vi "Inst.TC.Create.vi"(8 "error in (no error)":errorcluster, 11 "Inst.TC in":refnum<class "Inst.TC.lvclass">) -> (0 "error out":errorcluster, 2 "Inst.TC Public Events":T1, 3 "Inst.TC out":refnum<class "Inst.TC.lvclass">)   [LabVIEW 2019, in "Inst.TC.lvclass"]
uses:
  Inst.TC.lvclass
  C:/Program Files (x86)/National Instruments/LabVIEW 2019/user.lib/LevyLab/Instrument Framework/Instrument/Instrument.lvclass
  C:/Program Files (x86)/National Instruments/LabVIEW 2019/vi.lib/JKI/JKI SMO/SMO/SMO.lvclass
  Typedefs/PublicEvents--Cluster.ctl
  Typedefs/PublicEvents--Inst.TC.MessageFromProcess.ctl
  <userlib>/LevyLab/RemoteControl/RemoteControl/Typedefs/Message--Cluster.ctl
  <vilib>/JKI/JKI SMO/SMO/Typedefs/SMOState --Enum.ctl
  Inst.TC.lvclass/Inst.TC.ctl
  <vilib>/JKI/JKI SMO/SMO/SMO.lvclass
  <userlib>/LevyLab/Instrument Framework/Instrument/Instrument.lvclass
  FP-TC-Shared/FP-TC-Shared.lvclass
  <userlib>/LevyLab/RemoteControl/RemoteControl/RemoteControl.lvclass
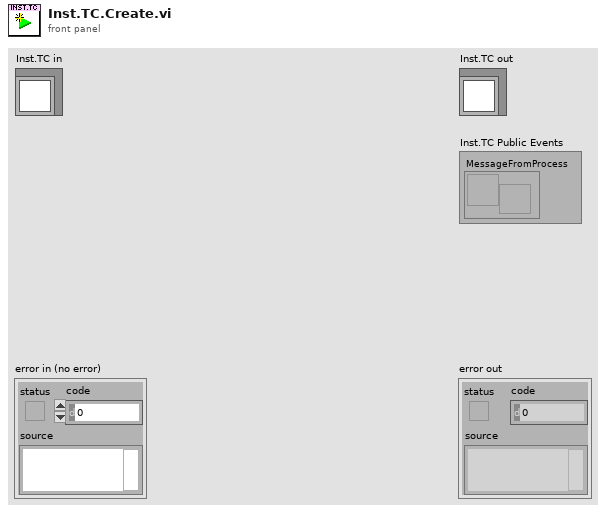
[diagram p1: front panel]
types:
  T1 = typedef "Inst.TC.lvclass/PublicEvents--Cluster.ctl" = cluster{"MessageFromProcess":refnum<user-event>}
  T2 = typedef "SMO.lvclass/SMOState --Enum.ctl" = enum16{"unknown", "Created", "Started", "Stopped"}
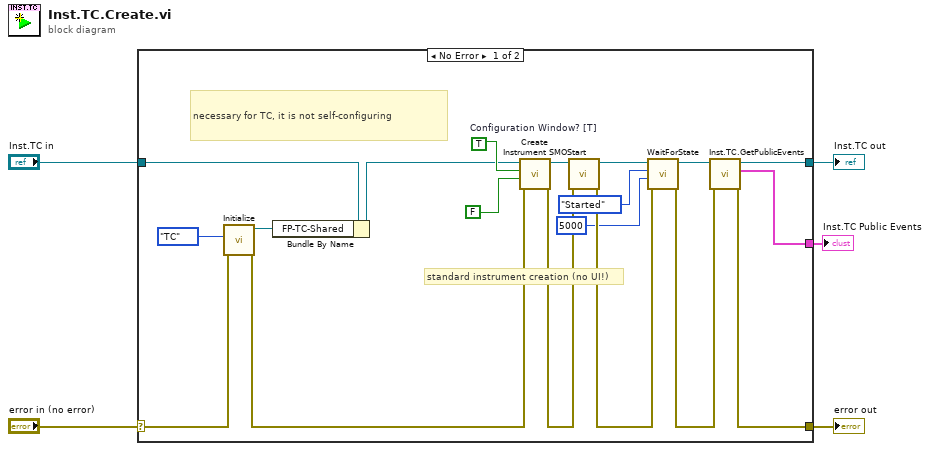
[diagram p0: block diagram]
diagram:
  n1 = case shown="No Error" "error in (no error)" {
    selector: "error in (no error)" -> [w10 w26]
    tunnel: [w15 w26] -> w4
    tunnel: [w14 w25] -> w2
    tunnel: "Inst.TC in" -> [w9 w25]
    tunnel: [w13 _] -> w1
    frame No Error {
      w20 = TRUE  # Configuration Window? [T]
      # "necessary for TC, it is not self-configuring"
      # "standard instrument creation (no UI!)"
      n2 = call "Initialize.vi"("error in (no error)"=w10, "Application"=enum16{"TC", "FP"}."TC") -> ("error out"=w7:errorcluster, "FP-TC-Shared out"=w11:refnum<class "FP-TC-Shared.lvclass">)  [unwired: 8 in]
      n3 = Bundle By Name(cluster=w9, "FP-TC-Shared"=w11) -> (w8:refnum<class "Inst.TC.lvclass">)
      n4 = call <userlib>:"Create Instrument SMO.vi"("error in (no error)"=w7, "Debug Mode? [F]"=FALSE, "Configuration Window? [T]"=w20, "Instrument in"=w8) -> ("error out"=w18:errorcluster, "Instrument out"=w19:refnum<class "Inst.TC.lvclass">)  [unwired: 6 in]
      n5 = call <vilib>:"Start.vi"("error in (no error)"=w18, "SMO"=w19) -> ("error out"=w24:errorcluster, "SMO out"=w22:refnum<class "Inst.TC.lvclass">)  [unwired: 8 in]
      n6 = call <vilib>:"WaitForState.vi"("error in (no error)"=w24, "timeout in ms (-1)"=5000, "State (unknown: any state)"=SMOState_--Enum."Started", "SMO in"=w22) -> ("error out"=w16:errorcluster, "SMO out"=w17:refnum<class "Inst.TC.lvclass">)  [unwired: 5 in, 1 out]
      n7 = call "Inst.TC.GetPublicEvents.vi"("error in (no error)"=w16, "Inst.TC in"=w17) -> ("error out"=w15:errorcluster, "Inst.TC Public Events"=w13:T1, "Inst.TC out"=w14:refnum<class "Inst.TC.lvclass">)  [unwired: 7 in]
    }
    frame Error {
    }
  }
  "error out" <- w4
  "Inst.TC out" <- w2
  "Inst.TC Public Events" <- w1
